vi "Test Scrollback Rotate.vi"() -> ()   [LabVIEW 2020, in "Terminal.lvlib" / "TermBuffer.lvclass"]
uses:
  TermBuffer.lvclass
panel:
  out "Buffer":string
  out "Scrollback":string
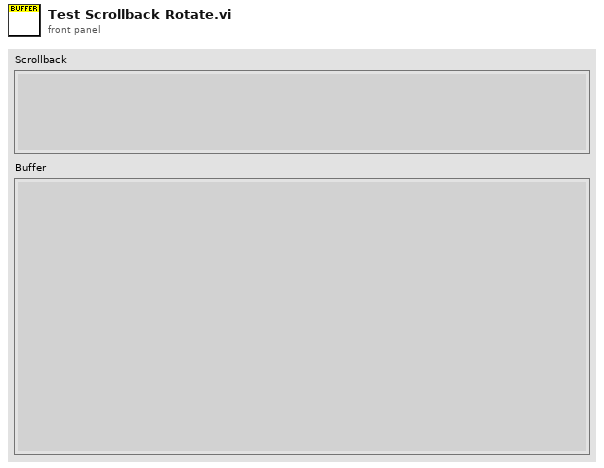
[diagram p1: front panel]
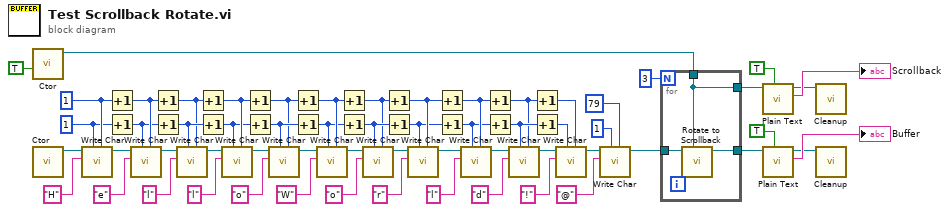
[diagram p0: block diagram]
diagram:
  w58 = 1 ("Col")
  w57 = 1 ("Row")
  n1 = call "Ctor.vi"("Is Scrollback? (F)"=TRUE) -> ("TermBuffer out"=w10:refnum<class "TermBuffer.lvclass">)  [unwired: 9 in, 1 out]
  n2 = call "Ctor.vi"() -> ("TermBuffer out"=w60:refnum<class "TermBuffer.lvclass">)  [unwired: 10 in, 1 out]
  n3 = call "Write Char.vi"("Col"=w58, "Row"=w57, "Char"="H", "TermBuffer in"=w60) -> ("TermBuffer out"=w56:refnum<class "TermBuffer.lvclass">)  [unwired: 6 in, 1 out]
  n4 = Increment(x=w58) -> (x+1=w43:i32)
  n5 = Increment(x=w57) -> (x+1=w42:i32)
  n6 = call "Write Char.vi"("Col"=w43, "Row"=w42, "Char"="e", "TermBuffer in"=w56) -> ("TermBuffer out"=w17:refnum<class "TermBuffer.lvclass">)  [unwired: 6 in, 1 out]
  n7 = Increment(x=w43) -> (x+1=w40:i32)
  n8 = Increment(x=w42) -> (x+1=w41:i32)
  n9 = call "Write Char.vi"("Col"=w40, "Row"=w41, "Char"="l", "TermBuffer in"=w17) -> ("TermBuffer out"=w18:refnum<class "TermBuffer.lvclass">)  [unwired: 6 in, 1 out]
  n10 = Increment(x=w40) -> (x+1=w39:i32)
  n11 = Increment(x=w41) -> (x+1=w38:i32)
  n12 = call "Write Char.vi"("Col"=w39, "Row"=w38, "Char"="l", "TermBuffer in"=w18) -> ("TermBuffer out"=w19:refnum<class "TermBuffer.lvclass">)  [unwired: 6 in, 1 out]
  n13 = Increment(x=w39) -> (x+1=w36:i32)
  n14 = Increment(x=w38) -> (x+1=w37:i32)
  n15 = call "Write Char.vi"("Col"=w36, "Row"=w37, "Char"="o", "TermBuffer in"=w19) -> ("TermBuffer out"=w20:refnum<class "TermBuffer.lvclass">)  [unwired: 6 in, 1 out]
  n16 = Increment(x=w36) -> (x+1=w35:i32)
  n17 = Increment(x=w37) -> (x+1=w34:i32)
  n18 = call "Write Char.vi"("Col"=w35, "Row"=w34, "Char"="W", "TermBuffer in"=w20) -> ("TermBuffer out"=w21:refnum<class "TermBuffer.lvclass">)  [unwired: 6 in, 1 out]
  n19 = Increment(x=w35) -> (x+1=w32:i32)
  n20 = Increment(x=w34) -> (x+1=w33:i32)
  n21 = call "Write Char.vi"("Col"=w32, "Row"=w33, "Char"="o", "TermBuffer in"=w21) -> ("TermBuffer out"=w22:refnum<class "TermBuffer.lvclass">)  [unwired: 6 in, 1 out]
  n22 = Increment(x=w32) -> (x+1=w31:i32)
  n23 = Increment(x=w33) -> (x+1=w30:i32)
  n24 = call "Write Char.vi"("Col"=w31, "Row"=w30, "Char"="r", "TermBuffer in"=w22) -> ("TermBuffer out"=w23:refnum<class "TermBuffer.lvclass">)  [unwired: 6 in, 1 out]
  n25 = Increment(x=w31) -> (x+1=w29:i32)
  n26 = Increment(x=w30) -> (x+1=w28:i32)
  n27 = call "Write Char.vi"("Col"=w29, "Row"=w28, "Char"="l", "TermBuffer in"=w23) -> ("TermBuffer out"=w24:refnum<class "TermBuffer.lvclass">)  [unwired: 6 in, 1 out]
  n28 = Increment(x=w29) -> (x+1=w26:i32)
  n29 = Increment(x=w28) -> (x+1=w27:i32)
  n30 = call "Write Char.vi"("Col"=w26, "Row"=w27, "Char"="d", "TermBuffer in"=w24) -> ("TermBuffer out"=w25:refnum<class "TermBuffer.lvclass">)  [unwired: 6 in, 1 out]
  n31 = Increment(x=w26) -> (x+1=w45:i32)
  n32 = Increment(x=w27) -> (x+1=w44:i32)
  n33 = call "Write Char.vi"("Col"=w45, "Row"=w44, "Char"="!", "TermBuffer in"=w25) -> ("TermBuffer out"=w16:refnum<class "TermBuffer.lvclass">)  [unwired: 6 in, 1 out]
  n34 = call "Write Char.vi"("Col"=79 ("Row"), "Row"=1, "Char"="@", "TermBuffer in"=w16) -> ("TermBuffer out"=w12:refnum<class "TermBuffer.lvclass">)  [unwired: 6 in, 1 out]
  n35 = for {
    N: 3 -> [_]
    tunnel: w12 -> [w63]
    tunnel: w10 -> [w62]
    tunnel: [w62] -> w8
    tunnel: [w61] -> w3
    n36 = call "Rotate to Scrollback.vi"("Scrollback"=w62, "TermBuffer in"=w63) -> ("TermBuffer out"=w61:refnum<class "TermBuffer.lvclass">)  [unwired: 8 in, 1 out]
  }
  n37 = call "Plain Text.vi"("Strip Line Ends? (F)"=TRUE, "TermBuffer in"=w8) -> ("Contents"=→"Scrollback":string, "TermBuffer out"=w2:refnum<class "TermBuffer.lvclass">)  [unwired: 7 in, 1 out]
  n38 = call "Plain Text.vi"("Strip Line Ends? (F)"=TRUE, "TermBuffer in"=w3) -> ("Contents"=→"Buffer":string, "TermBuffer out"=w1:refnum<class "TermBuffer.lvclass">)  [unwired: 7 in, 1 out]
  n39 = call "Cleanup.vi"("TermBuffer in"=w2) -> ()  [unwired: 10 in, 1 out]
  n40 = call "Cleanup.vi"("TermBuffer in"=w1) -> ()  [unwired: 10 in, 1 out]
